vi "Bury.vi"(8 "Error In":errorcluster, 11 "Selection List[]":refnum<vi>[](array[refnum])) -> (0 "Error Out":errorcluster, 3 "Change Made?":bool)   [LabVIEW 2017, in "Toolkit VIs.lvlib"]
doc: "Burys the corpse of legacy code. This removes the grave (Diagram Disable Structure) and leaves behind the Spirit frame, which should be enabled before burying the corpse. Note, the corpse frame will no longer exists and be pernamently deleted."
uses:
  Toolkit VIs.lvlib
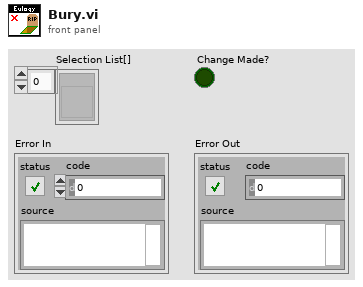
[diagram p1: front panel]
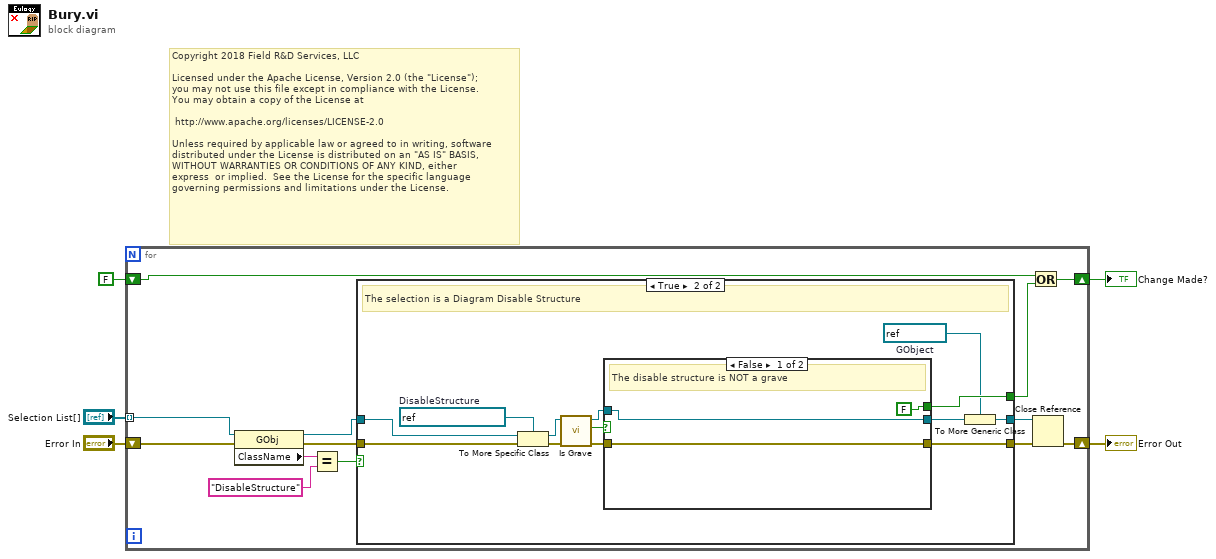
[diagram p0: block diagram]
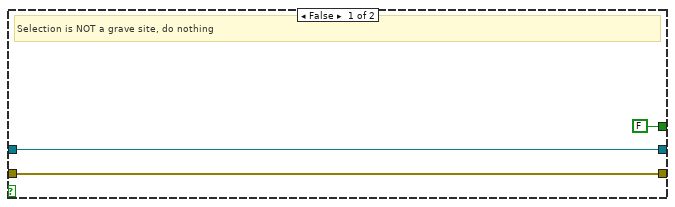
[diagram p2: hidden frame]
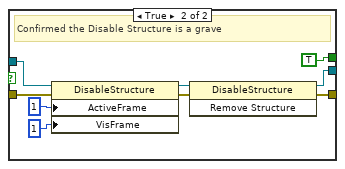
[diagram p3: hidden frame]
diagram:
  # "Copyright 2018 Field R&D Services, LLC\n\nLicensed under the Apache License, Version 2.0 (the \"License\");\nyou may not use this file except in compliance with the License.\nYou may obtain a copy of the License at\n\n\thttp://www.apache.org/licenses/LICENSE-2.0\n\nUnless required by applicable law or agreed to in writing, software\ndistributed under the License is distributed on an \"AS IS\" BASIS,\nWITHOUT WARRANTIES OR CONDITIONS OF ANY KIND, either \nexpress  or implied.  See the License for the specific language \ngoverning permissions and limitations under the License."
  n1 = for {
    shift-right: [w6] -> w5
    shift-left: "Error In" -> [w18]
    tunnel: "Selection List[]" -> [w12] mode=indexing
    shift-right: [w9] -> w3
    shift-left: FALSE -> [w11]
    n2 = property class="GObj"(reference=w12, error in=w18) -> (reference out=w14:refnum<vi>, error out=w13:errorcluster, "ClassName"=w17:string)
    n3 = Equal?(x=w17, y="DisableStructure") -> (x = y?=w15:bool)
    n4 = case shown="True" w15 {
      tunnel: w14 -> [w20 w33]
      tunnel: w13 -> [w19 w32]
      tunnel: [FALSE ("y") w30] -> w10
      tunnel: [w19 w29] -> w8
      tunnel: [w20 w22] -> w7
      frame False {
        # "Selection is NOT a grave site, do nothing"
      }
      frame True {
        w23 = refnum<vi> refnum  # GObject
        w34 = refnum<vi> refnum  # DisableStructure
        # "The selection is a Diagram Disable Structure"
        n5 = To More Specific Class(target class=w34, reference=w33, error in=w32) -> (specific class reference=w31:refnum<vi>, error out=w27:errorcluster)
        n6 = call "Is Grave.vi"("Error In"=w27, "DisableStructure In"=w31) -> ("Error Out"=w26:errorcluster, "Grave?"=w25:bool, "DisableStructure Out"=w28:refnum<vi>)  [unwired: 7 in]
        n7 = case shown="False" w25 {
          tunnel: [FALSE ("y") TRUE ("y")] -> w30
          tunnel: [w36 w39] -> w29
          tunnel: w28 -> [w35 w43]
          tunnel: w26 -> [w36 w42]
          tunnel: [w35 w38] -> w24
          frame False {
            # "The disable structure is NOT a grave"
          }
          frame True {
            # "Confirmed the Disable Structure is a grave"
            n8 = property class="DisableStructure"(reference=w43, error in=w42, "ActiveFrame"=i16 1 ("Active Frame"), "VisFrame"=u32 1 ("Visible Frame")) -> (reference out=w45:refnum<vi>, error out=w40:errorcluster)
            n9 = invoke class="DisableStructure" method="Remove Structure"(reference=w45, error in=w40) -> (reference out=w38:refnum<vi>, error out=w39:errorcluster)  [unwired: 1 in, 1 out]
          }
        }
        n10 = To More Generic Class(target class=w23, reference=w24) -> (generic class reference=w22:refnum<vi>)
      }
    }
    n11 = Or(x=w11, y=w10) -> (x .or. y?=w9:bool)
    n12 = Close Reference(reference=w7, error in (no error)=w8) -> (error out=w6:errorcluster)
  }
  "Error Out" <- w5
  "Change Made?" <- w3
